vi "MSEncoder Case-11-UpdRFChFunc.vi"(8 "error in (no error)":errorcluster, 9 "ParamValIn":variant, 11 "MSEncoder in":refnum<class "MSEncoder.lvclass">) -> (0 "error out":errorcluster, 3 "MSEncoder out":refnum<class "MSEncoder.lvclass">)   [LabVIEW 2018, in "MSEncoder.lvclass"]
uses:
  MSEncoder.lvclass
  Ctl/MSEditorParam updRFChFunc.ctl
  MSEncoder.lvclass/MSEncoder.ctl
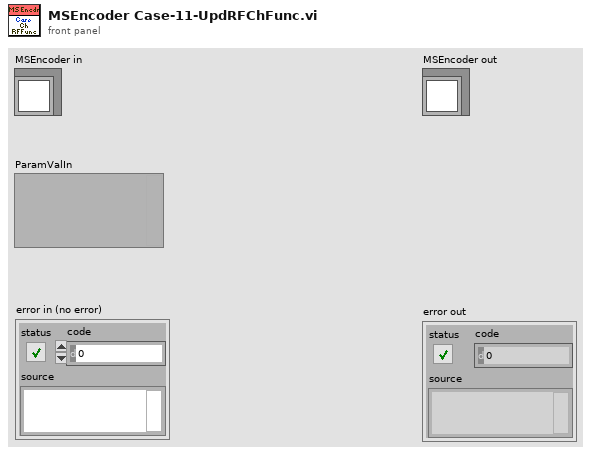
[diagram p1: front panel]
types:
  T1 = typedef "MSEditorParam updRFChFunc.ctl" = cluster{"ch1":u8, "ch2":u8, "ch3":u8}
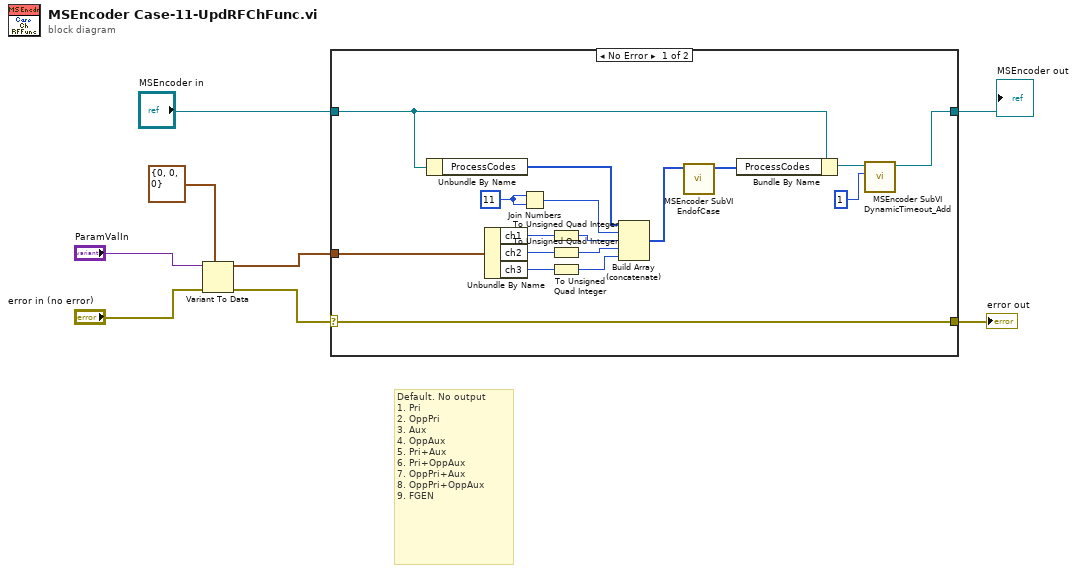
[diagram p0: block diagram]
diagram:
  # "Default. No output\n1. Pri\n2. OppPri\n3. Aux\n4. OppAux\n5. Pri+Aux\n6. Pri+OppAux\n7. OppPri+Aux\n8. OppPri+OppAux\n9. FGEN"
  n1 = Variant To Data(error in="error in (no error)", type=T1 {"ch1"=0, "ch2"=0, "ch3"=0} ("ParamValueType"), Variant="ParamValIn") -> (data=w3:T1, error out=w2:errorcluster)
  n2 = case shown="No Error" w2 {
    selector: w2 -> [w19 w27]
    tunnel: "MSEncoder in" -> [w24 w26]
    tunnel: [w19 w27] -> w8
    tunnel: [w16 w26] -> w7
    tunnel: w3 -> [w18 _]
    frame No Error {
      w22 = u32 11
      n3 = Unbundle By Name(w24) -> ("ProcessCodes"=w25:u64[])
      n4 = Unbundle By Name(w18) -> ("ch1"=w14:u8, "ch2"=w12:u8, "ch3"=w9:u8)
      n5 = Join Numbers(hi=w22, lo=w22) -> ((hi.lo)=w21:u64)
      n6 = To Unsigned Quad Integer(1:w14) -> (0:w13:u64)
      n7 = To Unsigned Quad Integer(1:w12) -> (0:w11:u64)
      n8 = To Unsigned Quad Integer(1:w9) -> (0:w10:u64)
      n9 = Build Array (concatenate)(w25, w21, w13, w11, w10) -> (w20:u64[])
      n10 = call "MSEncoder SubVI EndofCase.vi"("Case codes"=w20) -> ("Case codes with end"=w23:u64[])  [unwired: 9 in, 1 out]
      n11 = Bundle By Name(cluster=w24, "ProcessCodes"=w23) -> (w17:refnum<class "MSEncoder.lvclass">)
      n12 = call "MSEncoder SubVI DynamicTimeout_Add.vi"("Timeout_ms"=1, "MSEncoder"=w17) -> ("MSEncoder"=w16:refnum<class "MSEncoder.lvclass">)  [unwired: 8 in, 1 out]
    }
    frame Error {
    }
  }
  "error out" <- w8
  "MSEncoder out" <- w7
